vi "Create DVR_Notifier.vi"(11 "error in (no error)":errorcluster) -> (4 "data value reference":refnum<data-value>, 15 "error out":errorcluster)   [LabVIEW 2020, in "Notifiers.lvclass"]
doc: "Create Notifier object DVR."
uses:
  Classes/Children/Intra-Application/Children/With Data/Children/Notifiers/Notifiers.lvclass
  Classes/Children/Intra-Application/Children/With Data/Children/Notifiers/Notifiers.lvclass/Notifiers.ctl
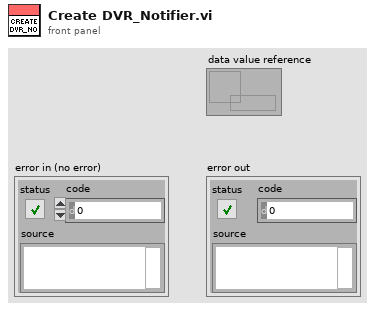
[diagram p1: front panel]
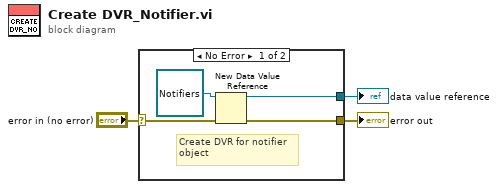
[diagram p0: block diagram]
diagram:
  n1 = case shown="No Error" "error in (no error)" {
    selector: "error in (no error)" -> [w6 w8]
    tunnel: [w5 w8] -> w2
    tunnel: [w4 _] -> w1
    frame No Error {
      # "Create DVR for notifier\nobject"
      n2 = New Data Value Reference(data value=refnum<class "Notifiers.lvclass"> refnum ("Data Communication Transmitter.lvlib:Notifiers.lvclass"), error in=w6) -> (data value reference=w4:refnum<data-value>, error out=w5:errorcluster)
    }
    frame Error {
    }
  }
  "error out" <- w2
  "data value reference" <- w1
